vi "myRIO v1.0 IRQ Info FGV.vi"(7 "Action":T1=enum."Set", 8 "error in (no error)":errorcluster, 11 "Generic IRQ Info in":T2) -> (0 "error out":errorcluster, 3 "Generic IRQ Info out":T2)   [LabVIEW 2021]
uses:
  <vilib>/myRIO/Common/Instrument Driver Framework/myRIO v1.0/IRQ/typedefs/Generic IRQ Array.ctl
  <vilib>/myRIO/Common/Instrument Driver Framework/myRIO v1.0/IRQ/typedefs/Generic IRQ.ctl
  <vilib>/myRIO/Common/Instrument Driver Framework/myRIO v1.0/IRQ/typedefs/IRQ Type.ctl
  <vilib>/myRIO/Common/Instrument Driver Framework/myRIO v1.0/IRQ/typedefs/IO IRQ Channels Enum.ctl
  <vilib>/myRIO/Common/Instrument Driver Framework/myRIO v1.0/IRQ/typedefs/Callback VI Ref.ctl
  <vilib>/myRIO/Common/Instrument Driver Framework/Utilities/typedefs/FPGA Ref Manager Action Enum.ctl
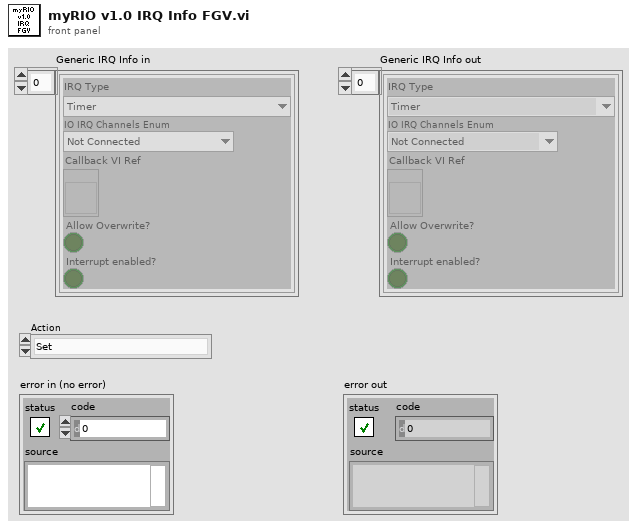
[diagram p1: front panel]
types:
  T1 = typedef "FPGA Ref Manager Action Enum.ctl" = enum16{"Get", "Set", "Reset"}
  T2 = typedef "Generic IRQ Array.ctl" = T3[]
  T3 = typedef "Generic IRQ.ctl" = cluster{"IRQ Type":T4, "IO IRQ Channels Enum":T5, "Callback VI Ref":T6, "Allow Overwrite?":bool, "Interrupt enabled?":bool}
  T4 = typedef "IRQ Type.ctl" = enum16{"Timer", "Analog falling edge", "Analog rising edge", "Digital falling edge", "Digital rising edge", "Digital edge"}
  T5 = typedef "IO IRQ Channels Enum.ctl" = enum16{"Not Connected", "A/AI0 (Interrupt)", "A/AI1 (Interrupt)", "A/DIO0 (Interrupt)", "A/DIO1 (Interrupt)", "A/DIO2 (Interrupt)", "A/DIO3 (Interrupt)", "Button0 (Interrupt)", "B/AI0 (Interrupt)", "B/AI1 (Interrupt)", "B/DIO0 (Interrupt)", "B/DIO1 (Interrupt)", "B/DIO2 (Interrupt)", "B/DIO3 (Interrupt)"}
  T6 = typedef "Callback VI Ref.ctl" = refnum<vi>
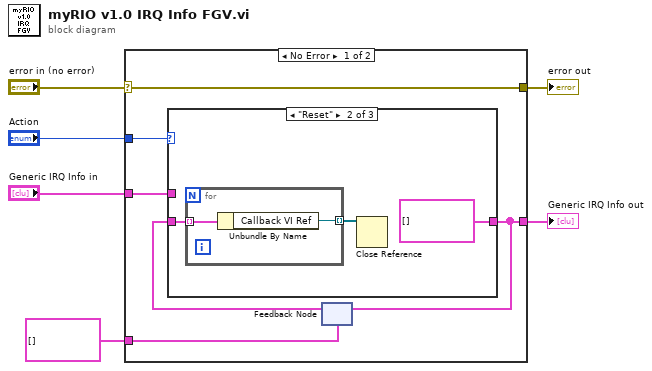
[diagram p0: block diagram]
diagram:
  n1 = case shown="No Error" "error in (no error)" {
    selector: "error in (no error)" -> [w8 w21]
    tunnel: "Action" -> [w12 _]
    tunnel: "Generic IRQ Info in" -> [w11 _]
    tunnel: [w10 w20] -> w4
    tunnel: [w8 w21] -> w2
    tunnel: T2 [] ("Interrupt Infos in") -> [w7 w20]
    frame No Error {
      n2 = feedback #1(w7) -> (w9:T2)
      n3 = case shown="\"Reset\"" w12 {
        tunnel: [w13 T2 [] ("Interrupt Infos in") w19] -> w10
        tunnel: w11 -> [_ _ w19]
        tunnel: w9 -> [w13 w14 _]
        frame "Get", Default {
        }
        frame "Reset" {
          n4 = for {
            tunnel: w14 -> [w18] mode=indexing
            tunnel: [w17] -> w15 mode=indexing
            n5 = Unbundle By Name(w18) -> ("Callback VI Ref"=w17:T6)
          }
          n6 = Close Reference(reference=w15) -> ()  [unwired: 1 in, 1 out]
        }
        frame "Set" {
        }
      }
      n7 = feedback-in #1(w10) -> ()
    }
    frame Error {
    }
  }
  "Generic IRQ Info out" <- w4
  "error out" <- w2
